vi "USB2XXX_LIN_Test.vi"() -> ()   [LabVIEW 2010]
uses:
  PublicFiles/USB2XXX.dll
panel:
  out "write return":i32
  out "pLINMsg out":T1
  out "read return":i32
  in  "pLINWiteMsg":T1
  in  "pConfig":T2
  in  "Channel Index":u8(ring) items=["CH0"]
  in  "Device Index":i32(ring) items=["0", "1", "2", "3", "4", "5"]
  out "Flag(T:Write;F:Read)":bool=TRUE
  in  "stop":bool
  in  "Read":bool
  in  "Write":bool
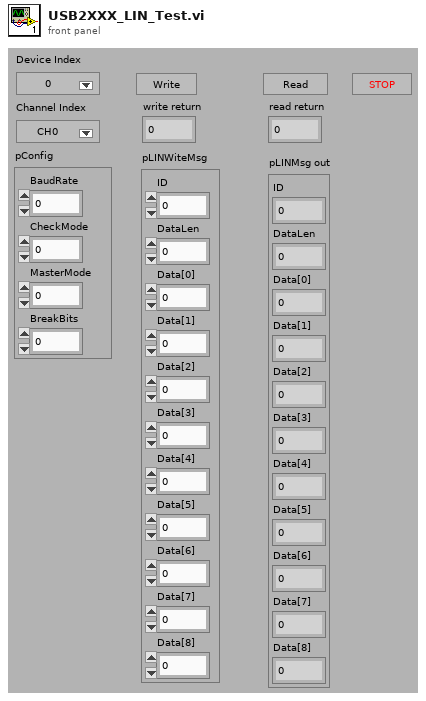
[diagram p1: front panel]
types:
  T1 = cluster{"ID":u8, "DataLen":u8, "Data[0]":u8, "Data[1]":u8, "Data[2]":u8, "Data[3]":u8, "Data[4]":u8, "Data[5]":u8, "Data[6]":u8, "Data[7]":u8, "Data[8]":u8}
  T2 = cluster{"BaudRate":u32, "CheckMode":u8, "MasterMode":u8, "BreakBits":u8}
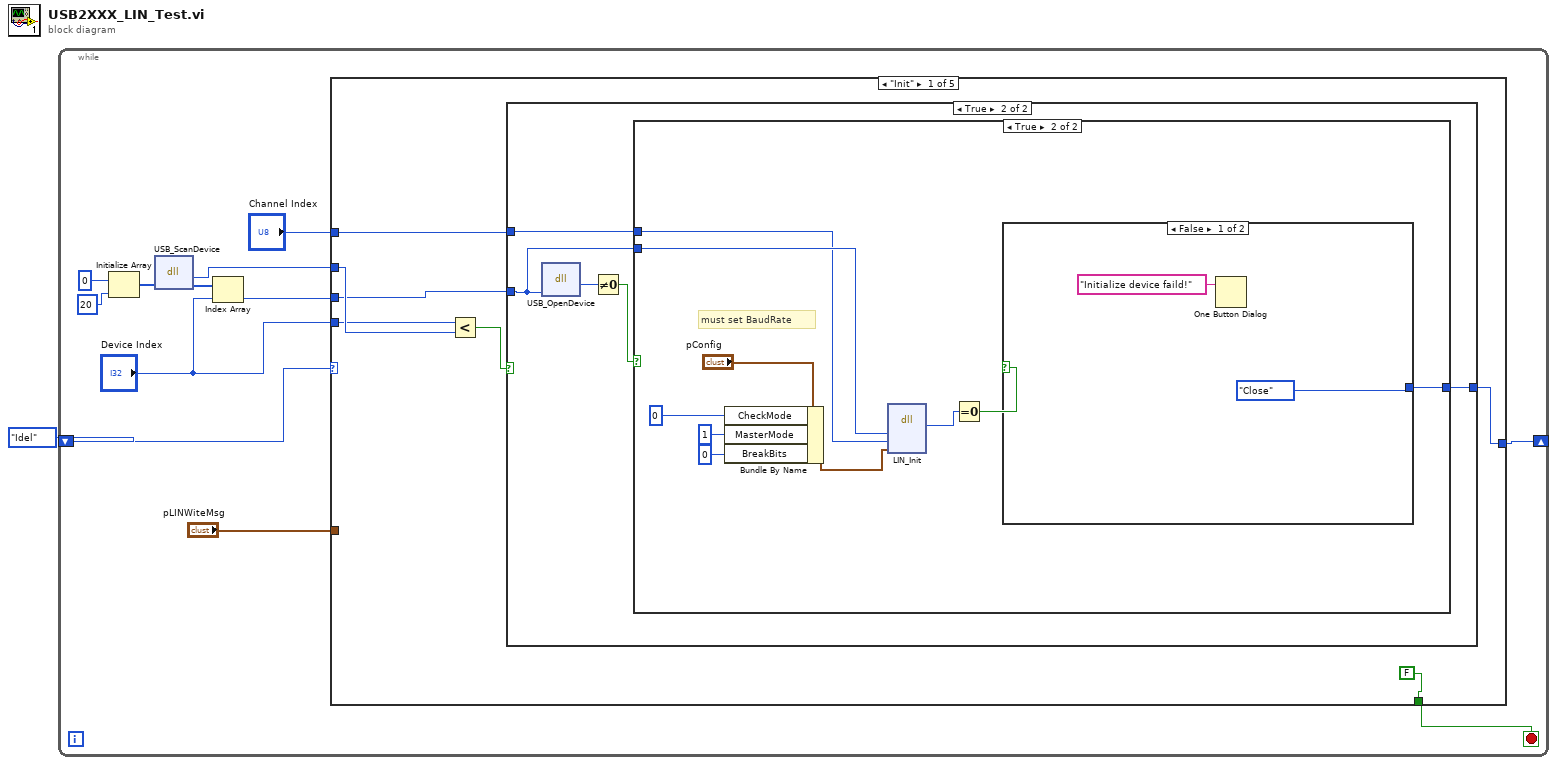
[diagram p0: block diagram]
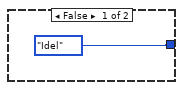
[diagram p2: hidden frame]
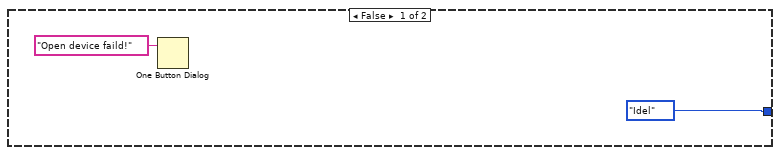
[diagram p3: hidden frame]
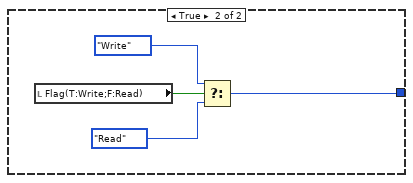
[diagram p4: hidden frame]
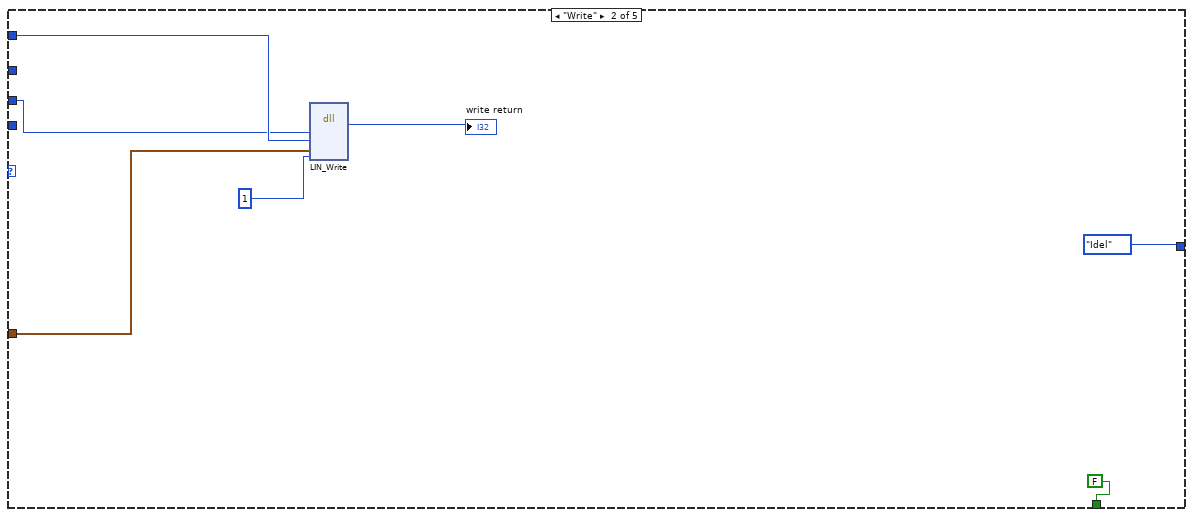
[diagram p5: hidden frame]
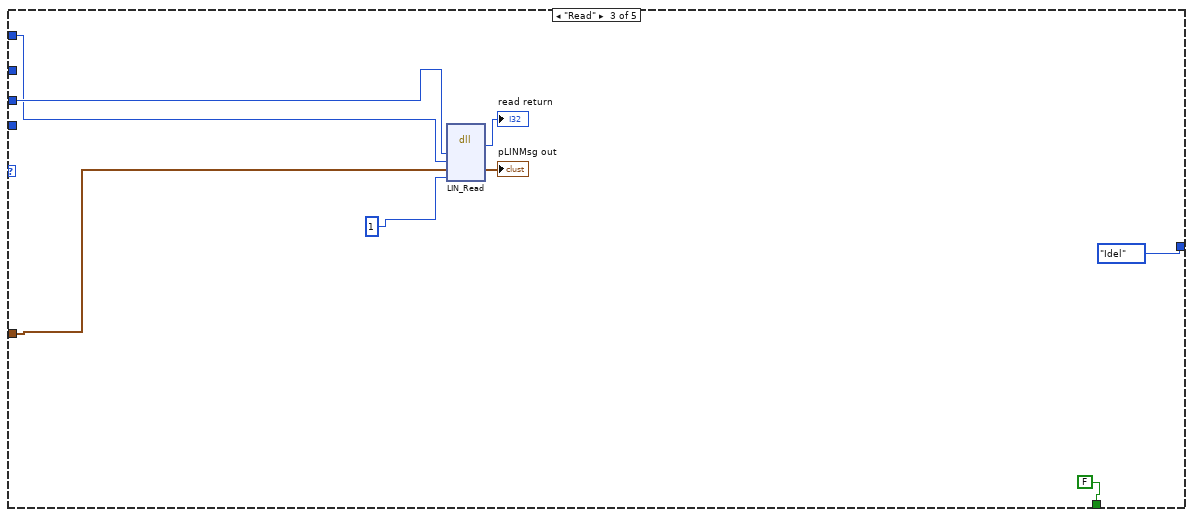
[diagram p6: hidden frame]
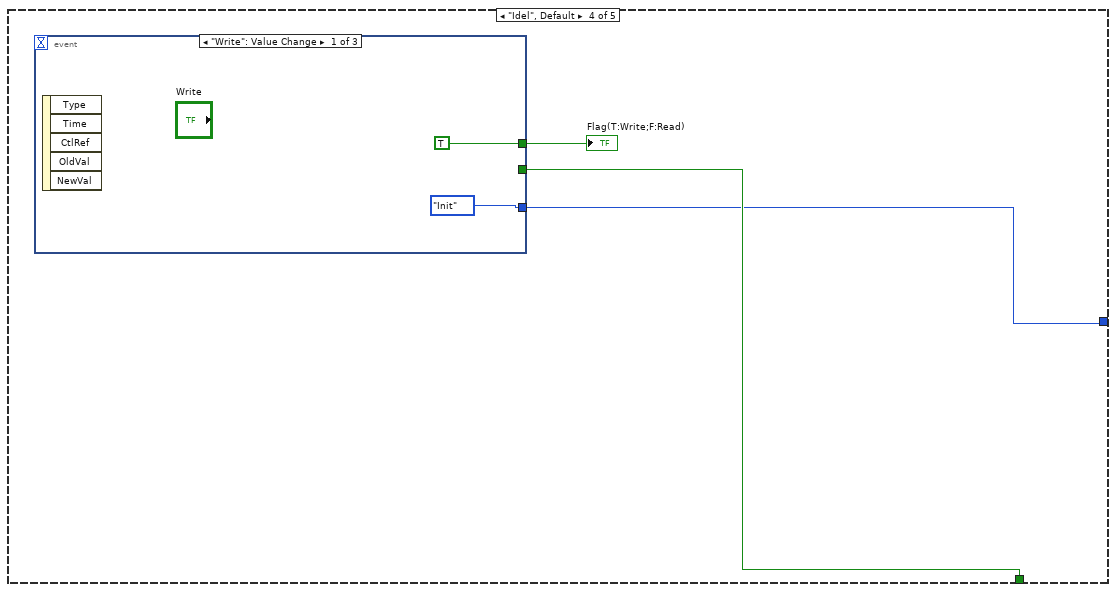
[diagram p7: hidden frame]
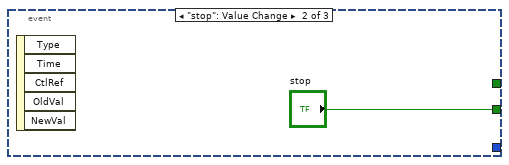
[diagram p8: hidden frame]
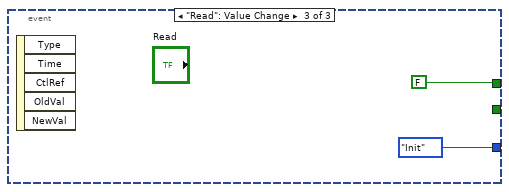
[diagram p9: hidden frame]
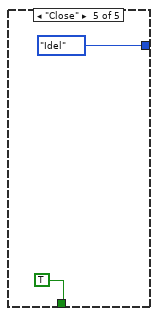
[diagram p10: hidden frame]
diagram:
  n1 = while {
    shift-right: [w12] -> _
    shift-left: enum16{"Init", "Write", "Read", "Idel", "Close"}."Idel" ("Enum") -> [w13]
    stop <- w10 stop-if-true
    n2 = Initialize Array(0, 20 ("dimension size")) -> (w9:i32[])
    n3 = dll-call lib="F:/OtherWork/STM32/USB2XXX_Example/trunk/Labview/PublicFiles/USB2XXX.*" fn="USB_ScanDevice"("pDevNum"=w9) -> ("return type"=w4:i32, "pDevNum"=w6:i32[])  [unwired: 3 in, 2 out]
    n4 = Index Array(array=w6, index="Device Index") -> (element=w5:i32)
    n5 = case shown="\"Init\"" w13 {
      tunnel: [w19 enum16{"Init", "Write", "Read", "Idel", "Close"}."Idel" ("Enum") enum16{"Init", "Write", "Read", "Idel", "Close"}."Idel" ("Enum") w60 enum16{"Init", "Write", "Read", "Idel", "Close"}."Idel" ("Enum")] -> w12
      tunnel: w5 -> [w15 w47 w55 _ _]
      tunnel: "Channel Index" -> [w18 w48 w54 _ _]
      tunnel: [FALSE FALSE FALSE w61 TRUE] -> w10
      tunnel: w4 -> [w16 _ _ _ _]
      tunnel: "Device Index" -> [w14 _ _ _ _]
      tunnel: "pLINWiteMsg" -> [_ w46 w53 _ _]
      frame "Init" {
        n6 = Less?(x=w14, y=w16) -> (x < y?=w20:bool)
        n7 = case shown="True" w20 {
          tunnel: w15 -> [_ w23]
          tunnel: w18 -> [_ w24]
          tunnel: [enum16{"Init", "Write", "Read", "Idel", "Close"}."Idel" ("Enum") w22] -> w19
          frame False {
          }
          frame True {
            n8 = dll-call lib="F:/OtherWork/STM32/USB2XXX_Example/trunk/Labview/PublicFiles/USB2XXX.*" fn="USB_OpenDevice"("DevIndex"=w23) -> (w26:u8)  [unwired: 4 in, 2 out]
            n9 = Not Equal To 0?(x=w26) -> (x != 0?=w25:bool)
            n10 = case shown="True" w25 {
              tunnel: w24 -> [_ w31]
              tunnel: w23 -> [_ w32]
              tunnel: [enum16{"Init", "Write", "Read", "Idel", "Close"}."Idel" ("Enum") w34] -> w22
              frame False {
                n11 = One Button Dialog(message="Open device faild!") -> ()  [unwired: 1 in, 1 out]
              }
              frame True {
                # "must set BaudRate"
                n12 = Bundle By Name(cluster="pConfig", "CheckMode"=u16 0 ("OwnAddr"), "MasterMode"=u8 1 ("Master"), "BreakBits"=u8 0 ("AddrBits")) -> (w30:T2)
                n13 = dll-call lib="F:/OtherWork/STM32/USB2XXX_Example/trunk/Labview/PublicFiles/USB2XXX.*" fn="LIN_Init"("DevHandle"=w32, "LINIndex"=w31, "pConfig"=w30) -> (w29:i32)  [unwired: 6 in, 2 out]
                n14 = Equal To 0?(x=w29) -> (x = 0?=w35:bool)
                n15 = case shown="False" w35 {
                  tunnel: [enum16{"Init", "Write", "Read", "Idel", "Close"}."Close" ("Enum") w41] -> w34
                  frame False {
                    n16 = One Button Dialog(message="Initialize device faild!") -> ()  [unwired: 1 in, 1 out]
                  }
                  frame True {
                    n17 = local read "Flag(T:Write;F:Read)"() -> (w44:bool)
                    n18 = Select(t=enum16{"Init", "Write", "Read", "Idel", "Close"}."Write" ("Enum"), s=w44, f=enum16{"Init", "Write", "Read", "Idel", "Close"}."Read" ("Enum")) -> (s? t:f=w41:enum16{"Init", "Write", "Read", "Idel", "Close"})
                  }
                }
              }
            }
          }
        }
      }
      frame "Write" {
        n19 = dll-call lib="F:/OtherWork/STM32/USB2XXX_Example/trunk/Labview/PublicFiles/USB2XXX.*" fn="LIN_Write"("DevHandle"=w47, "LINIndex"=w48, "pLINMsg"=w46, "Len"=u32 1) -> (→"write return":i32)  [unwired: 7 in, 2 out]
      }
      frame "Read" {
        n20 = dll-call lib="F:/OtherWork/STM32/USB2XXX_Example/trunk/Labview/PublicFiles/USB2XXX.*" fn="LIN_Read"("DevHandle"=w55, "LINIndex"=w54, "pLINMsg"=w53, "Len"=u32 1) -> (→"read return":i32, "pLINMsg"=→"pLINMsg out":T1)  [unwired: 6 in, 2 out]
      }
      frame "Idel", Default {
        n21 = event shown="[0] \"Write\": Value Change" {
          selector: _ -> [_ _ _]
          dyn-events: _ -> [_ _ _]
          timeout: _ -> [_ _ _]
          tunnel: [TRUE _ FALSE] -> w62
          tunnel: [_ "stop" _] -> w61
          tunnel: [enum16{"Init", "Write", "Read", "Idel", "Close"}."Init" ("Enum") _ enum16{"Init", "Write", "Read", "Idel", "Close"}."Init" ("Enum")] -> w60
          event "Write": Value Change {
            n22 = event-data() -> ()  [unwired: 1 in, 5 out]
          }
          event "stop": Value Change {
            n23 = event-data() -> ()  [unwired: 1 in, 5 out]
          }
          event "Read": Value Change {
            n24 = event-data() -> ()  [unwired: 1 in, 5 out]
          }
        }
        "Flag(T:Write;F:Read)" <- w62
      }
      frame "Close" {
      }
    }
  }
